vi "setAxisGrids.vi"(8 "DrawZeroAxes":T1, 9 "Minor Gridlines":T1, 10 "Major Gridlines":T1, 11 "String in":string) -> (2 "command":string, 3 "String out":string)   [LabVIEW 2012]
uses:
  gridlines.ctl
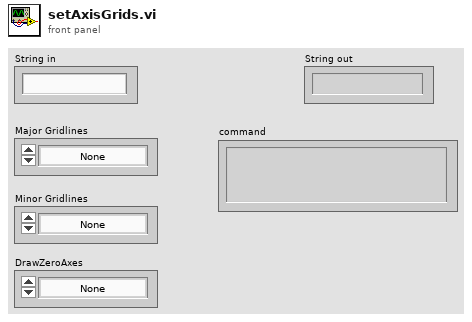
[diagram p1: front panel]
types:
  T1 = typedef "gridlines.ctl" = enum16{"None", "X only", "Y only", "Both X and Y"}
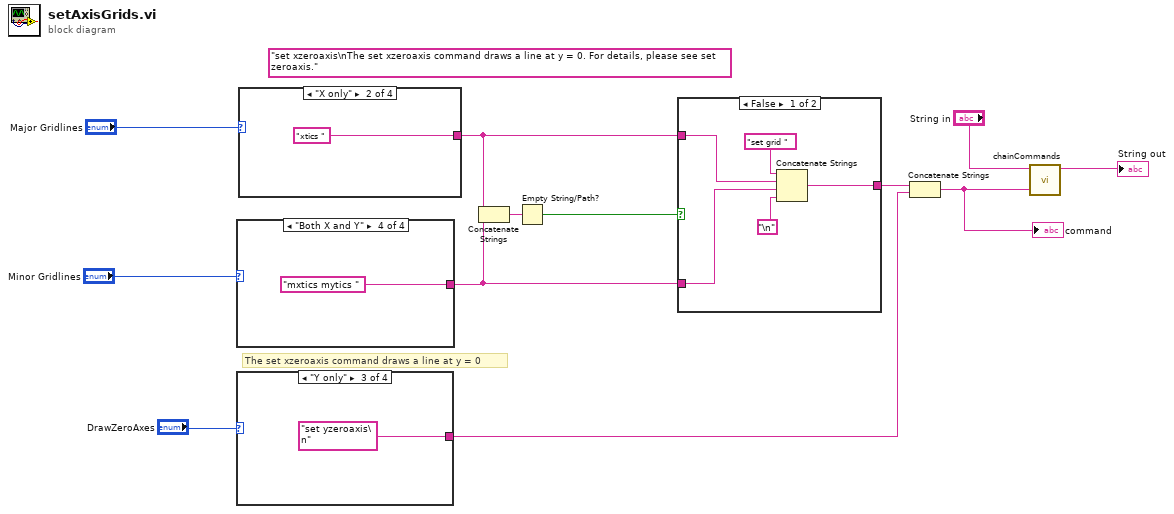
[diagram p0: block diagram]
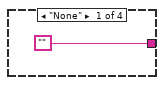
[diagram p2: hidden frame]
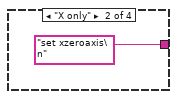
[diagram p3: hidden frame]
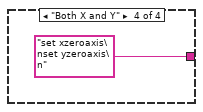
[diagram p4: hidden frame]
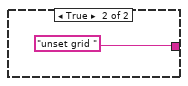
[diagram p5: hidden frame]
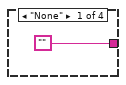
[diagram p6: hidden frame]
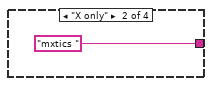
[diagram p7: hidden frame]
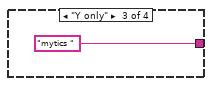
[diagram p8: hidden frame]
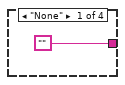
[diagram p9: hidden frame]
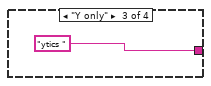
[diagram p10: hidden frame]
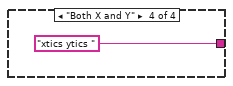
[diagram p11: hidden frame]
diagram:
  (unwired) "set xzeroaxis\nThe set xzeroaxis command draws a line at y = 0. For details, please see set zeroaxis."
  # "The set xzeroaxis command draws a line at y = 0"
  n1 = case shown="\"Both X and Y\"" "Minor Gridlines" {
    tunnel: ["" "mxtics " "mytics " "mxtics mytics "] -> w12
    frame "None" {
    }
    frame "X only" {
    }
    frame "Y only" {
    }
    frame "Both X and Y" {
    }
  }
  n2 = case shown="\"Y only\"" "DrawZeroAxes" {
    tunnel: ["" "set xzeroaxis\n" "set yzeroaxis\n" "set xzeroaxis\nset yzeroaxis\n"] -> w1
    frame "None" {
    }
    frame "X only" {
    }
    frame "Y only" {
    }
    frame "Both X and Y" {
    }
  }
  n3 = case shown="\"X only\"" "Major Gridlines" {
    tunnel: ["" "xtics " "ytics " "xtics ytics "] -> w11
    frame "None" {
    }
    frame "X only" {
    }
    frame "Y only" {
    }
    frame "Both X and Y" {
    }
  }
  n4 = Concatenate Strings(w11, w12) -> (w9:string)
  n5 = Empty String/Path?(string/path=w9) -> (empty?=w10:bool)
  n6 = case shown="False" w10 {
    tunnel: [w28 "unset grid "] -> w4
    tunnel: w11 -> [w27 _]
    tunnel: w12 -> [w26 _]
    frame False {
      n7 = Concatenate Strings("set grid ", w27, w26, "\n") -> (w28:string)
    }
    frame True {
    }
  }
  n8 = Concatenate Strings(w4, w1) -> (w2:string)
  "command" <- w2
  n9 = call "chainCommands.vi"("Command"=w2, "StringIn"="String in") -> ("StringOut"=→"String out":string)  [unwired: 9 in]
